vi "enableSCurve.vi"(0 "ACESDEController in":refnum<class "ACESDEController.lvclass">, 2 "axis (nc - for use only with multi-axis applications)":T1, 5 "error in (no error)":errorcluster) -> (14 "ACESDEController out":refnum<class "ACESDEController.lvclass">, 17 "success?":bool, 18 "response":string, 19 "error out":errorcluster)   [LabVIEW 2020, in "classes.lvlib" / "ACESDEController.lvclass"]
uses:
  ACESDEController.lvclass
  C:/GEECS/Developers Version/source/Device Drivers/Newmark-NSC-A/Arcus Driver 3.0.0/ArcusUsbComm/classes/Controller/_Controller.lvclass
  common/controls/axis.ctl
  Controller/_Controller.lvclass
  libraries/common.lvlib
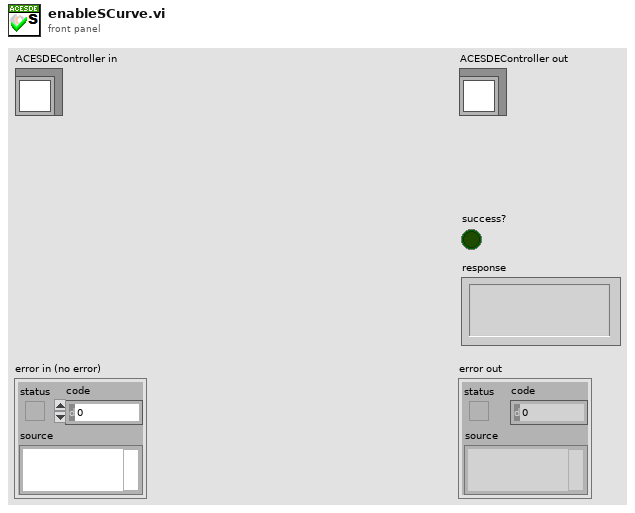
[diagram p1: front panel]
types:
  T1 = typedef "common.lvlib/axis.ctl" = enum16{"X", "Y", "Z", "U"}
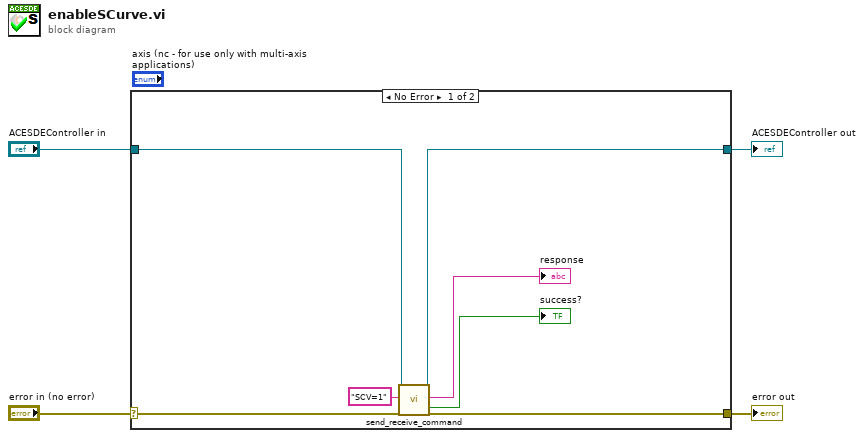
[diagram p0: block diagram]
diagram:
  n1 = case shown="No Error" "error in (no error)" {
    selector: "error in (no error)" -> [w9 w13]
    tunnel: [w8 w13] -> w3
    tunnel: [w6 w12] -> w1
    tunnel: "ACESDEController in" -> [w7 w12]
    frame No Error {
      n2 = call "send_receive_command.vi"("reference (in)"=w7, "ASCII Command (in)"="SCV=1", "error in (no error)"=w9) -> ("reference (out)"=w6:refnum<class "ACESDEController.lvclass">, "response (out)"=→"response":string, "success?"=→"success?":bool, "error out"=w8:errorcluster)  [unwired: 12 in, 1 out]
    }
    frame Error {
    }
  }
  "error out" <- w3
  "ACESDEController out" <- w1
